vi "TangoGroupWriteAttributeTest.vi"() -> ()   [LabVIEW 2013, in "examples.lvlib"]
uses:
  examples.lvlib
  vis/lv-2013/tango_vi.llb/fromDoubleScalar.vi
  vis/lv-2013/tango_vi.llb/tango.lvlib
panel:
  out "T.Grp.W Error":errorcluster
  out "attribute to write on the group":string="double_scalar"
  in  "value for dev-1 in the group":dbl=1.1
  in  "value for dev-2 in the group":dbl=2.2
  in  "value for dev-3 in the group":dbl=3.3
  in  "ignored devices":string[](array[string])
  in  "managed devices":string[](array[string])=["tango/tangotest/1", "tango/tangotest/2", "tango/tangotest/3"]
  in  "group name":string="w_test_group"
  out "group id":i32
  # "In this example we write a specific value on each device in the group"
  # "TANGO  Binding for LabVIEW - WriteAttributes example"
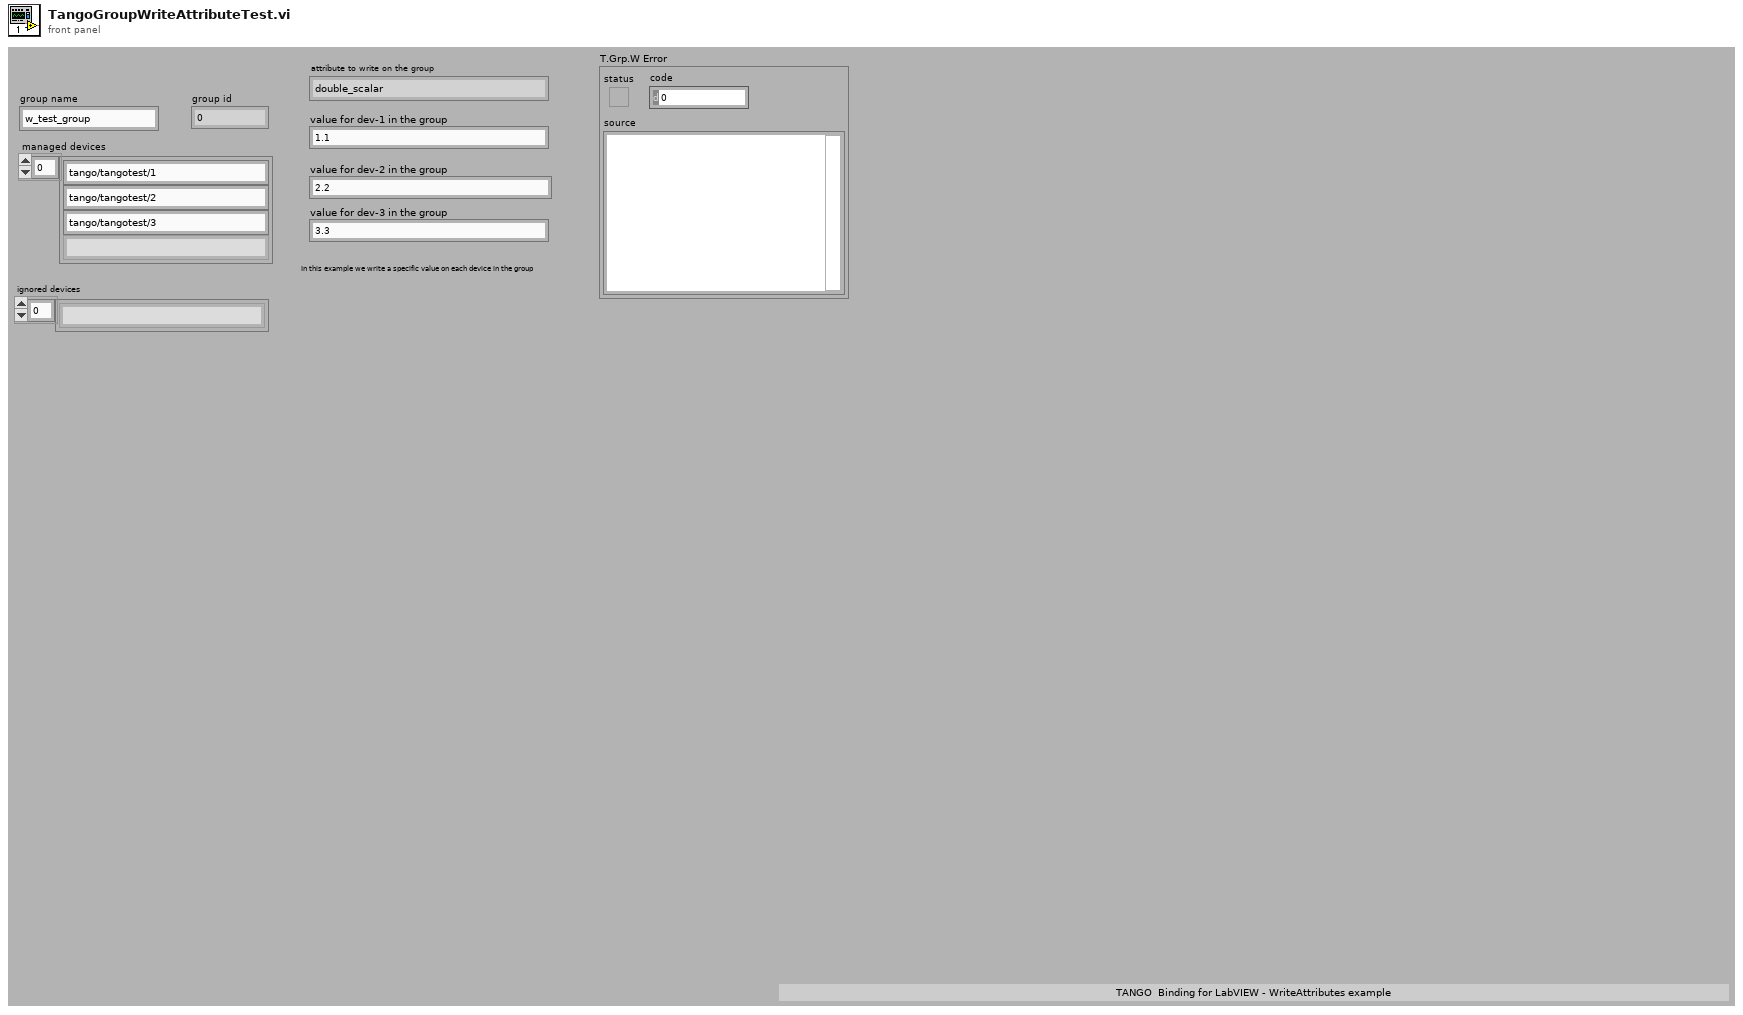
[diagram p1: front panel]
types:
  T1 = cluster{"device name":string, "attribute name":string, "quality value":i16, "quality string":string, "timestamp":dbl, "dim. x":i32, "dim. y":i32, "value":u8[], "error code":i32, "error stack":string[], "data type":u16}
  T2 = cluster{"device name":string, "attribute name":string, "quality value":i16, "quality string":string, "timestamp":dbl, "dim. x":i32, "dim. y":i32, "value":u8[], "error code":i32, "error stack":string[], "data type":u16}[]
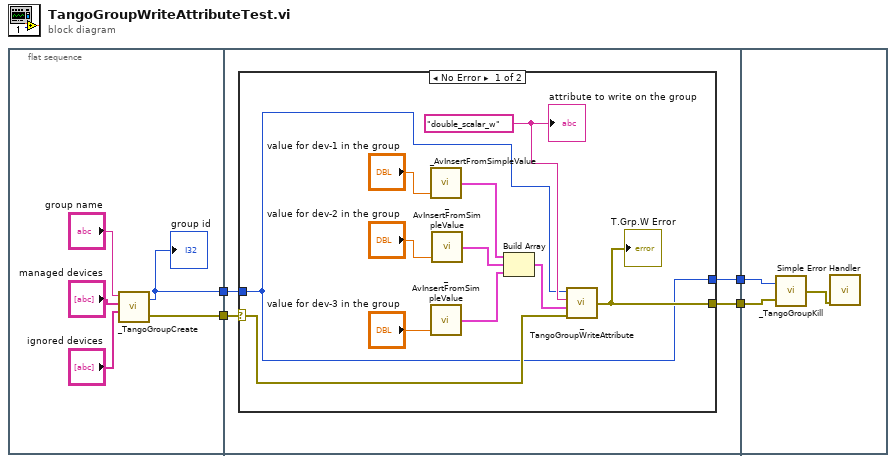
[diagram p0: block diagram]
diagram:
  n1 = flat-sequence {
    tunnel: [w8] -> w4
    tunnel: [w7] -> w3
    tunnel: w4 -> [w11]
    tunnel: [w10] -> w2
    tunnel: w3 -> [w13]
    tunnel: [w12] -> w1
    tunnel: w2 -> [w29]
    tunnel: w1 -> [w28]
    frame #0 {
      n2 = call "_TangoGroupCreate.vi"("ignored devices"="ignored devices", "managed devices"="managed devices", "group name"="group name") -> ("error out"=w7:errorcluster, "group id"=w8:i32)  [unwired: 1 in]
      "group id" <- w8
    }
    frame #1 {
      n3 = case shown="No Error" w13 {
        selector: w13 -> [w19 w26]
        tunnel: w11 -> [w15 w25]
        tunnel: [w20 w26] -> w12
        tunnel: [w15 w25] -> w10
        frame No Error {
          w21 = "double_scalar_w" ("attribute name")
          n4 = call-poly "_AvInsertFromSimpleValue.vi"("value"="value for dev-1 in the group") -> ("attribute value"=w17:T1)  [unwired: 2 in]
          n5 = call-poly "_AvInsertFromSimpleValue.vi"("value"="value for dev-3 in the group") -> ("attribute value"=w16:T1)  [unwired: 2 in]
          n6 = call-poly "_AvInsertFromSimpleValue.vi"("value"="value for dev-2 in the group") -> ("attribute value"=w18:T1)  [unwired: 2 in]
          n7 = Build Array(w17, w18, w16) -> (w14:T2)
          n8 = call "_TangoGroupWriteAttribute.vi"("error in"=w19, "values"=w14, "attribute name"=w21, "group id"=w15) -> ("error out"=w20:errorcluster)
          "T.Grp.W Error" <- w20
          "attribute to write on the group" <- w21
        }
        frame Error {
        }
      }
    }
    frame #2 {
      n9 = call "_TangoGroupKill.vi"("error in"=w28, "group id"=w29) -> ("error out"=w27:errorcluster)
      n10 = call <vilib>:"Simple Error Handler.vi"("error in (no error)"=w27) -> ()  [unwired: 4 in, 5 out]
    }
  }
